vi "globalSetUp.vi"(8 "error in (no error)":errorcluster, 11 "testcase-CSMResponse in":refnum<class "testcase-CSMResponse.lvclass">) -> (0 "error out":errorcluster, 3 "testcase-CSMResponse out":refnum<class "testcase-CSMResponse.lvclass">)   [LabVIEW 2017, in "testcase-CSMResponse.lvclass"]
uses:
  testcase-CSMResponse.lvclass
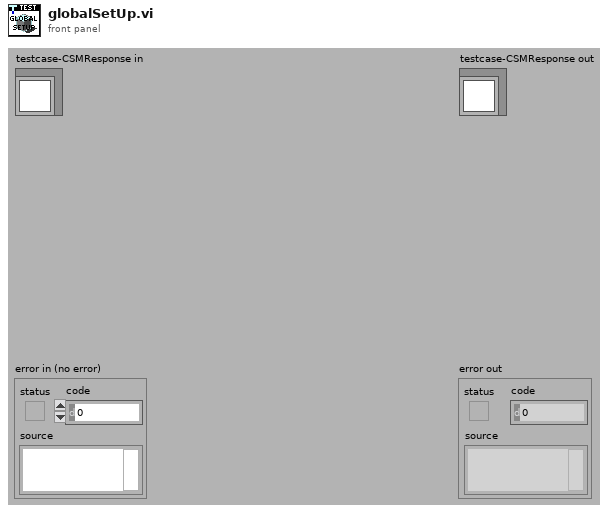
[diagram p1: front panel]
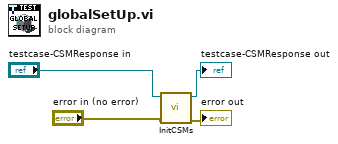
[diagram p0: block diagram]
diagram:
  n1 = call "InitCSMs.vi"("error in"="error in (no error)", "testcase-CSMResponse.lvclass in"="testcase-CSMResponse in") -> ("error out"=→"error out":errorcluster, "testcase-CSMResponse.lvclass out"=→"testcase-CSMResponse out":refnum<class "testcase-CSMResponse.lvclass">)  [unwired: 8 in]
